vi "Global - Channel.vi"() -> ()   [LabVIEW 2019]
uses:
  UDP - Event.ctl
  UDP - Status.ctl
panel:
  in  "Data":T3(array[cluster]) {"Status" items=["Stop", "Ramp Up", "Ramp Down", "Jog Up", "Jog Down", "PID Mode", "PID Ramp"]; "Event" items=["Stop", "Running", "PID", "Up Limit", "Down Limit", "Load Limit"]}
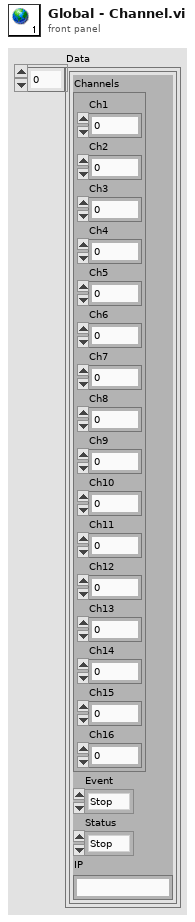
[diagram p1: front panel]
types:
  T1 = typedef "UDP - Event.ctl" = u16
  T2 = typedef "UDP - Status.ctl" = u16
  T3 = cluster{"Channels":cluster{"Ch1":sgl, "Ch2":sgl, "Ch3":sgl, "Ch4":sgl, "Ch5":sgl, "Ch6":sgl, "Ch7":sgl, "Ch8":sgl, "Ch9":sgl, "Ch10":sgl, "Ch11":sgl, "Ch12":sgl, "Ch13":sgl, "Ch14":sgl, "Ch15":sgl, "Ch16":sgl}, "Event":T1, "Status":T2, "IP":string}[]
diagram:
